vi "MS Initialization v2.vi"(6 "PID Cluster":T2={"L1 to L4 PID Cluster"={"L1 PID Gains"={"Kp"=0.005, "Kd"=0.5, "Ki"=0.0005}, "L2 PID Gains"={"Kp"=0.01, "Kd"=1.0, "Ki"=0.005}, "L3 PID Gains"={"Kp"=0.05, "Kd"=1.0, "Ki"=0.0005}, "L4 PID Gains"={"Kp"=0.1, "Kd"=0.1, "Ki"=0.0005}}, "Stage PID Cluster"={"Stage Z PID"={"Kp"=0.0005, "Kd"=0.001, "Ki"=0.0}, "Stage Y PID"={"Kp"=0.0003, "Kd"=0.01, "Ki"=0.0}, "Stage X PID"={"Kp"=0.0003, "Kd"=0.01, "Ki"=0.0}}, "OCT Z PID Gains"={"Kp"=0.0003, "Kd"=0.0001, "Ki"=0.01}}, 8 "error in":errorcluster, 9 "Offset Home 2 RCM":dbl[](array[numeric])=[0.0, 0.0, 0.0, 0.0], 10 "Prev Posit Cluster":T3={"Prev L1 to L4 Posit"=[0.0, 0.0, 0.0, 0.0], "Prev Stage Posit"=[6.0, 6.0, 6.0], "Prev OCT Z Posit"=0.0}, 11 "FPGA VI Reference In":refnum<k20>) -> (0 "error out":errorcluster, 2 "Last Posit Cluster":T1={"Last L1 to L4 Posit"=[0.0, 0.0, 0.0, 0.0], "Last Stage Posit"=[6.0, 6.0, 6.0], "Last OCT Z Posit"=0.0}, 3 "FPGA VI Reference Out":refnum<k20>)   [LabVIEW 2016]
uses:
  <vilib>/Platform/TimedLoop/XDataNode/timing_clust.ctl
  <vilib>/Platform/TimedLoop/XDataNode/nitl_modes.ctl
  <vilib>/Platform/TimedLoop/XDataNode/wakeup.ctl
  Global Variables.vi
  <vilib>/platform/TimedLoop/XDataNode/XDataNode.xnode
  <vilib>/Platform/TimedLoop/XDataNode/XDNodeRunTimeDep.lvlib
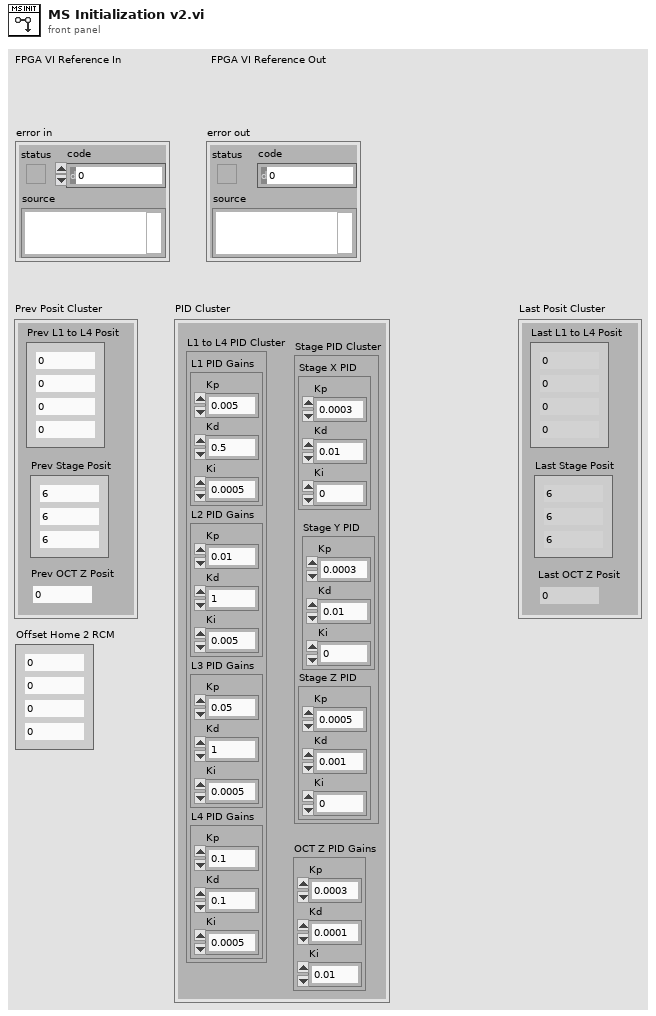
[diagram p1: front panel]
types:
  T1 = cluster{"Last L1 to L4 Posit":dbl[], "Last Stage Posit":dbl[], "Last OCT Z Posit":dbl}
  T2 = cluster{"L1 to L4 PID Cluster":cluster{"L1 PID Gains":cluster{"Kp":dbl, "Kd":dbl, "Ki":dbl}, "L2 PID Gains":cluster{"Kp":dbl, "Kd":dbl, "Ki":dbl}, "L3 PID Gains":cluster{"Kp":dbl, "Kd":dbl, "Ki":dbl}, "L4 PID Gains":cluster{"Kp":dbl, "Kd":dbl, "Ki":dbl}}, "Stage PID Cluster":cluster{"Stage Z PID":cluster{"Kp":dbl, "Kd":dbl, "Ki":dbl}, "Stage Y PID":cluster{"Kp":dbl, "Kd":dbl, "Ki":dbl}, "Stage X PID":cluster{"Kp":dbl, "Kd":dbl, "Ki":dbl}}, "OCT Z PID Gains":cluster{"Kp":dbl, "Kd":dbl, "Ki":dbl}}
  T3 = cluster{"Prev L1 to L4 Posit":dbl[], "Prev Stage Posit":dbl[], "Prev OCT Z Posit":dbl}
  T4 = typedef "XDNodeRunTimeDep.lvlib/timing_clust.ctl" = cluster{"Expected End [f-1]":u64, "Actual End [f-1]":u64, "Finished Late? [f-1]":bool, "Expected End [i-1]":u64, "Actual End [i-1]":u64, "Finished Late? [i-1]":bool, "Expected Start [i]":u64, "Actual Start [i]":u64, "Expected Start [f]":u64, "Actual Start [f]":u64, "Source Name":string, "Structure Name":string, "Period":i64, "Deadline":i64, "Offset":i64, "Start":i64, "Priority":i32, "Timeout":i32, "Mode":T5, "Wakeup Reason":T6, "Error":errorcluster, "Source Type":string, "Secondary Source Type":string, "Global End Time":u64, "Global Start Time":u64, "Frame Duration":u64, "Iteration Duration":u64, "Assigned CPU":i32, "I/O Scan Engine Mode":u32}
  T5 = typedef "XDNodeRunTimeDep.lvlib/nitl_modes.ctl" = enum32{"No Change", "Process missed periods, maintain original phase", "Discard missed periods, maintain original phase", "Process missed periods, ignore original phase", "Discard missed periods, ignore original phase"}
  T6 = typedef "XDNodeRunTimeDep.lvlib/wakeup.ctl" = enum32{"Normal", "Aborted", "Asynchronous wakeup", "Timing source error", "Timed loop error", "Timeout"}
  T7 = cluster{"L1 PID Gains":cluster{"Kp":dbl, "Kd":dbl, "Ki":dbl}, "L2 PID Gains":cluster{"Kp":dbl, "Kd":dbl, "Ki":dbl}, "L3 PID Gains":cluster{"Kp":dbl, "Kd":dbl, "Ki":dbl}, "L4 PID Gains":cluster{"Kp":dbl, "Kd":dbl, "Ki":dbl}}
  T8 = cluster{"Stage Z PID":cluster{"Kp":dbl, "Kd":dbl, "Ki":dbl}, "Stage Y PID":cluster{"Kp":dbl, "Kd":dbl, "Ki":dbl}, "Stage X PID":cluster{"Kp":dbl, "Kd":dbl, "Ki":dbl}}
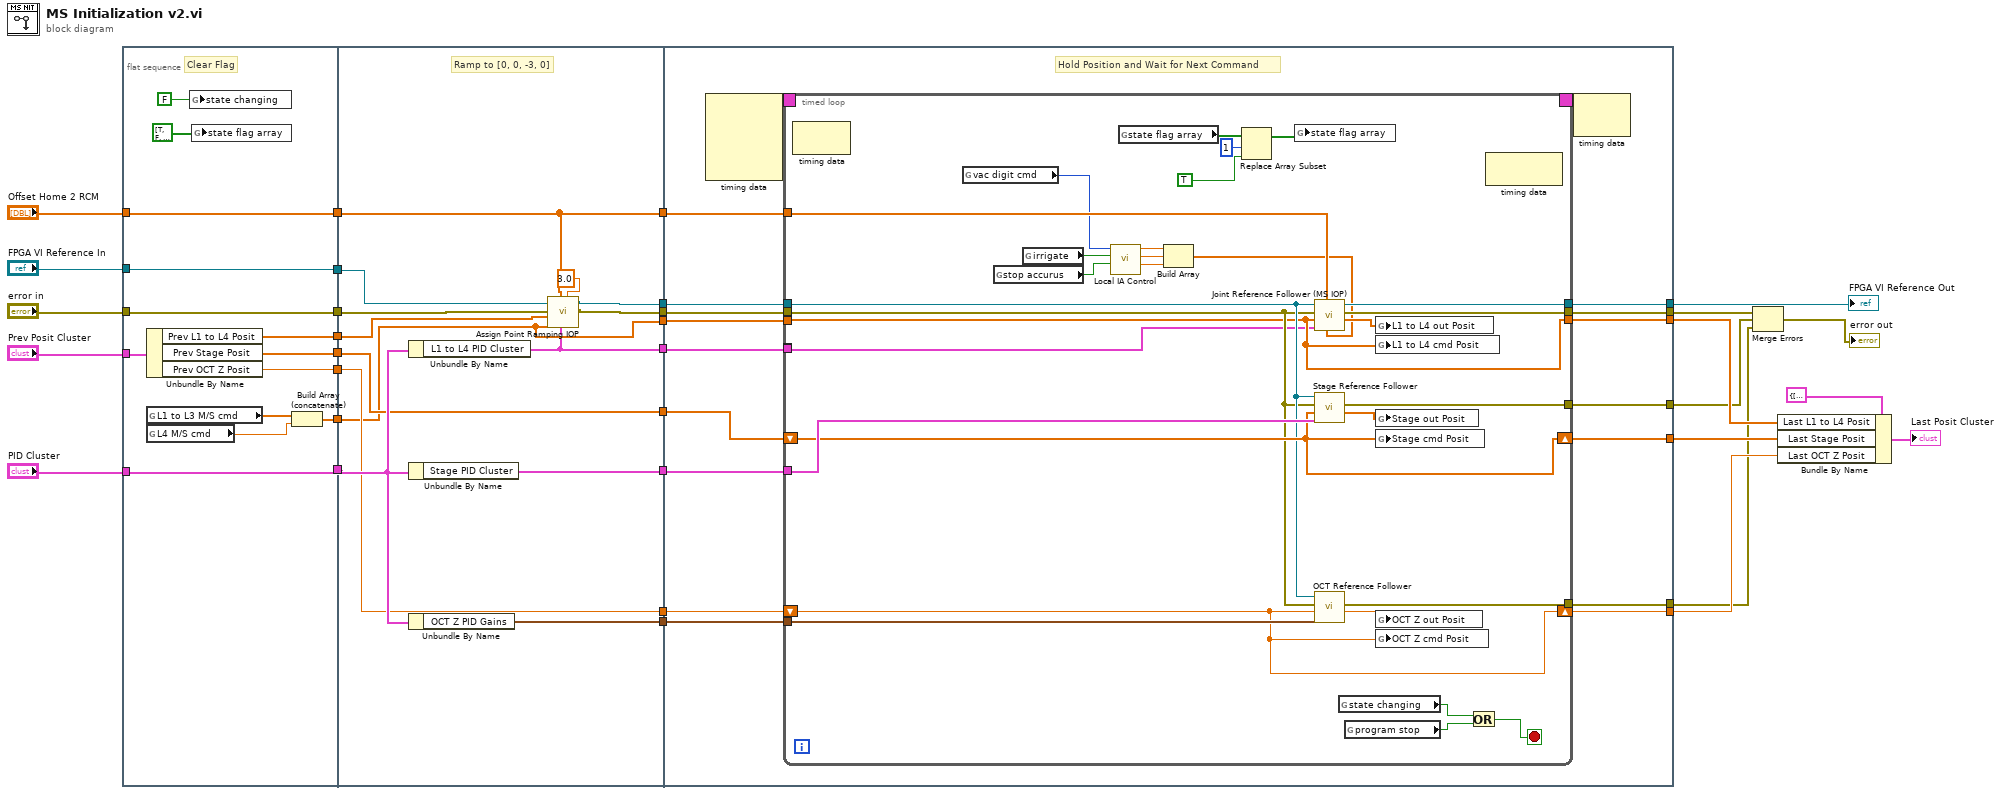
[diagram p0: block diagram]
diagram:
  n1 = flat-sequence {
    tunnel: "Prev Posit Cluster" -> [w43]
    tunnel: [w33] -> w31
    tunnel: [w42] -> w30
    tunnel: [w41] -> w29
    tunnel: "PID Cluster" -> [w41]
    tunnel: "error in" -> [w40]
    tunnel: [w40] -> w26
    tunnel: "Offset Home 2 RCM" -> [w39]
    tunnel: [w39] -> w24
    tunnel: [w38] -> w23
    tunnel: "FPGA VI Reference In" -> [w38]
    tunnel: [w37] -> w4
    tunnel: [w36] -> w2
    tunnel: w31 -> [w49]
    tunnel: w30 -> [w50]
    tunnel: w29 -> [w59]
    tunnel: w26 -> [w51]
    tunnel: w24 -> [w54]
    tunnel: w23 -> [w52]
    tunnel: [w47] -> w21
    tunnel: [w48] -> w20
    tunnel: [w46] -> w19
    tunnel: [w58] -> w18
    tunnel: [w57] -> w17
    tunnel: [w49] -> w16
    tunnel: [w54] -> w15
    tunnel: w4 -> [w56]
    tunnel: [w56] -> w3
    tunnel: w2 -> [w55]
    tunnel: [w55] -> w1
    tunnel: w21 -> [w75]
    tunnel: w20 -> [w74]
    tunnel: w19 -> [w73]
    tunnel: w18 -> [w72]
    tunnel: w17 -> [w71]
    tunnel: w16 -> [w70]
    tunnel: w15 -> [w69]
    tunnel: [w68] -> w14
    tunnel: [w67] -> w8
    tunnel: [w66] -> w11
    tunnel: [w65] -> w10
    tunnel: [w64] -> w9
    tunnel: [w63] -> w6
    tunnel: [w62] -> w5
    tunnel: w3 -> [w61]
    tunnel: w1 -> [w60]
    frame #0 {
      # "Clear Flag"
      n2 = Unbundle By Name(w43) -> ("Prev L1 to L4 Posit"=w42:dbl[], "Prev Stage Posit"=w37:dbl[], "Prev OCT Z Posit"=w36:dbl)
      n3 = global read "Global Variables.vi" "L1 to L3 M/S cmd"() -> (w35:dbl[])
      n4 = global read "Global Variables.vi" "L4 M/S cmd"() -> (w34:dbl)
      n5 = global write "Global Variables.vi" "state changing"(FALSE ("state changing")) -> ()
      n6 = global write "Global Variables.vi" "state flag array"(bool[] [TRUE, FALSE, FALSE, FALSE, FALSE, FALSE, FALSE, FALSE, FALSE] ("state flag array")) -> ()
      n7 = Build Array (concatenate)(w35, w34) -> (w33:dbl[])
    }
    frame #1 {
      # "Ramp to [0, 0, -3, 0]"
      n8 = Unbundle By Name(w59) -> ("L1 to L4 PID Cluster"=w46:T7)
      n9 = Unbundle By Name(w59) -> ("Stage PID Cluster"=w58:T8)
      n10 = Unbundle By Name(w59) -> ("OCT Z PID Gains"=w57:cluster{"Kp":dbl, "Kd":dbl, "Ki":dbl})
      n11 = call "Assign Point Ramping IOP.vi"("Ramp Time [sec]"=3.0, "L1 to L4 PID Cluster"=w46, "Offset Home2RCM"=w54, "Destination Posit Array [mm]"=w49, "Previous Posit Array"=w50, "error in"=w51, "FPGA VI Reference In"=w52) -> ("error out"=w48:errorcluster, "FPGA VI Reference Out"=w47:refnum<k20>)  [unwired: 2 in, 1 out]
    }
    frame #2 {
      # "Hold Position and Wait for Next Command"
      n12 = node-c288() -> (w77:T4)  [unwired: 4 in]
      n13 = timed-loop {
        timing: w77 -> [_]
        timing-out: [_] -> w76
        tunnel: w75 -> [w88]
        tunnel: w74 -> [w87]
        tunnel: [w85] -> _
        tunnel: w73 -> [w85]
        tunnel: w72 -> [w100]
        tunnel: w71 -> [w99]
        tunnel: w70 -> [w86]
        tunnel: w69 -> [w92]
        tunnel: [w91] -> w68
        tunnel: [w90] -> w67
        tunnel: [w86] -> w66
        tunnel: [w96] -> w63
        tunnel: [w95] -> w62
        shift-right: [w94] -> w65
        shift-left: w61 -> [w94]
        shift-right: [w93] -> w64
        shift-left: w60 -> [w93]
        stop <- w107 stop-if-true
        n14 = node-c288() -> ()  [unwired: 1 in, 1 out]
        n15 = global read "Global Variables.vi" "vac digit cmd"() -> (w78:i8)
        n16 = global read "Global Variables.vi" "stop accurus"() -> (w81:bool)
        n17 = global read "Global Variables.vi" "irrigate"() -> (w80:bool)
        n18 = call "Local IA Control.vi"("E-Stop Vacuum"=w81, "Irrigate?"=w80, "8bit integer"=w78) -> ("Accurus Engaged Vout"=w84:dbl, "Accurus ChB Vout"=w83:dbl, "Accurus ChA Vout"=w82:dbl)  [unwired: 6 in]
        n19 = global read "Global Variables.vi" "state flag array"() -> (w104:bool[])
        n20 = Build Array(w82, w83, w84) -> (w79:dbl[])
        n21 = Replace Array Subset(array=w104, new element=TRUE ("new element/subarray"), index=1) -> (w103:bool[])
        n22 = global write "Global Variables.vi" "state flag array"(w103) -> ()
        n23 = call "Joint Reference Follower (MS IOP).vi"("Acc Ctrl Array"=w79, "Offset Home2RCM [deg/mm]"=w92, "PID Ctrl Cluster"=w85, "Ref Array [deg/mm]"=w86, "error in"=w87, "FPGA VI Reference In"=w88) -> ("Output Posit Array [deg/mm]"=w89:dbl[], "error out"=w90:errorcluster, "FPGA VI Reference Out"=w91:refnum<k20>)  [unwired: 3 in]
        n24 = call "Stage Reference Follower.vi"("Stage PID Cluster"=w100, "Stage cmd Posit [mm]"=w94, "error in"=w87, "FPGA VI Reference In"=w88) -> ("Stage out Posit [mm]"=w98:dbl[], "error out"=w96:errorcluster)  [unwired: 5 in, 1 out]
        n25 = call "OCT Reference Follower.vi"("OCT Z PID Gains"=w99, "OCT  Z cmd Posit [mm]"=w93, "error in"=w87, "FPGA VI Reference In"=w88) -> ("OCT  Z out Posit [mm]"=w97:dbl, "error out"=w95:errorcluster)  [unwired: 5 in, 1 out]
        n26 = global read "Global Variables.vi" "state changing"() -> (w106:bool)
        n27 = global read "Global Variables.vi" "program stop"() -> (w105:bool)
        n28 = global write "Global Variables.vi" "L1 to L4 out Posit"(w89) -> ()
        n29 = global write "Global Variables.vi" "L1 to L4 cmd Posit"(w86) -> ()
        n30 = global write "Global Variables.vi" "Stage out Posit"(w98) -> ()
        n31 = global write "Global Variables.vi" "Stage cmd Posit"(w94) -> ()
        n32 = global write "Global Variables.vi" "OCT Z out Posit"(w97) -> ()
        n33 = global write "Global Variables.vi" "OCT Z cmd Posit"(w93) -> ()
        n34 = Or(x=w106, y=w105) -> (x .or. y?=w107:bool)
        n35 = node-c288() -> ()  [unwired: 1 in, 1 out]
      }
      n36 = node-c288(w76) -> ()  [unwired: 1 out]
    }
  }
  n37 = Merge Errors(w8, w6, w5) -> (→"error out":errorcluster)
  n38 = Bundle By Name(cluster=T1 {"Last L1 to L4 Posit"=[0.0, 0.0, 0.0, 0.0], "Last Stage Posit"=[6.0, 6.0, 6.0], "Last OCT Z Posit"=0.0} ("Last Posit Cluster 2"), "Last L1 to L4 Posit"=w11, "Last Stage Posit"=w10, "Last OCT Z Posit"=w9) -> (→"Last Posit Cluster":T1)
  "FPGA VI Reference Out" <- w14
